vi "Indirect FF PID Control.vi"(9 "Setpoint":dbl format="%#_13g", 11 "Parameter":i32) -> (3 "Indirect FF":bool)   [LabVIEW 2013]
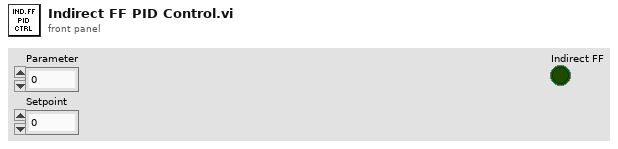
[diagram p1: front panel]
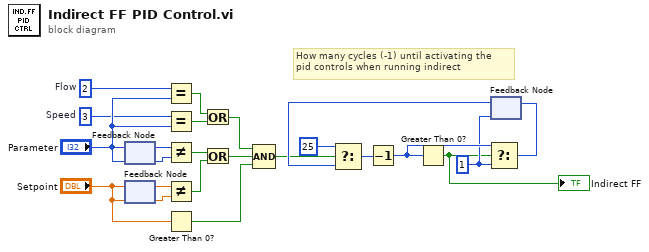
[diagram p0: block diagram]
diagram:
  w13 = 3  # Speed
  w14 = 2  # Flow
  w17 = 1
  # "How many cycles (-1) until activating the\npid controls when running indirect"
  n1 = feedback-in #1("Parameter") -> ()
  n2 = feedback #1("Parameter") -> (w19:i32)
  n3 = feedback #2("Setpoint") -> (w20:dbl)
  n4 = feedback-in #2("Setpoint") -> ()
  n5 = Equal?(x=w14, y="Parameter") -> (x = y?=w11:bool)
  n6 = Equal?(x=w13, y="Parameter") -> (x = y?=w12:bool)
  n7 = Not Equal?(x=w19, y="Parameter") -> (x != y?=w5:bool)
  n8 = Not Equal?(x=w20, y="Setpoint") -> (x != y?=w6:bool)
  n9 = Greater Than 0?(x="Setpoint") -> (x > 0?=w4:bool)
  n10 = Or(x=w11, y=w12) -> (x .or. y?=w3:bool)
  n11 = Or(x=w5, y=w6) -> (x .or. y?=w2:bool)
  n12 = Compound Arithmetic op=AND(w3, w2, w4) -> (w1:bool)
  n13 = feedback #3(w17) -> (w7:i32)
  n14 = Select(t=25, s=w1, f=w7) -> (s? t:f=w8:i32)
  n15 = Decrement(x=w8) -> (x-1=w18:i32)
  n16 = Greater Than 0?(x=w18) -> (x > 0?=w10:bool)
  "Indirect FF" <- w10
  n17 = Select(t=w18, s=w10, f=w17) -> (s? t:f=w9:i32)
  n18 = feedback-in #3(w9) -> ()
